vi "SystemeinstellungenV2_Screenshots.vi"(8 "error in":errorcluster, 11 "Screenshots Pfad":path) -> (0 "error out 2":errorcluster caption="error out", 3 "Screenshots Pfad  2":path caption="Screenshots Pfad")   [LabVIEW 2020, in "Backup.lvlib"]
uses:
  Backup.lvlib
  Seiten/System Einstellungen V2/System und Gaseinstellung V2.vi
  Seiten/System Einstellungen V2/System Einstellungen V2.lvlib
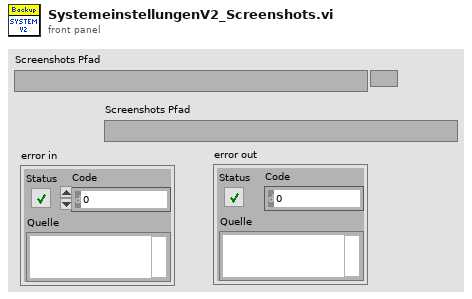
[diagram p1: front panel]
types:
  T1 = enum32{"Bad", "Idle", "Run top level", "Running"}
  T2 = typedef "imagedata.ctl" = cluster{"image type":i32, "image depth":i32, "image":u8[], "mask":u8[], "colors":u32[], "Rectangle":cluster{"left":i16, "top":i16, "right":i16, "bottom":i16}}
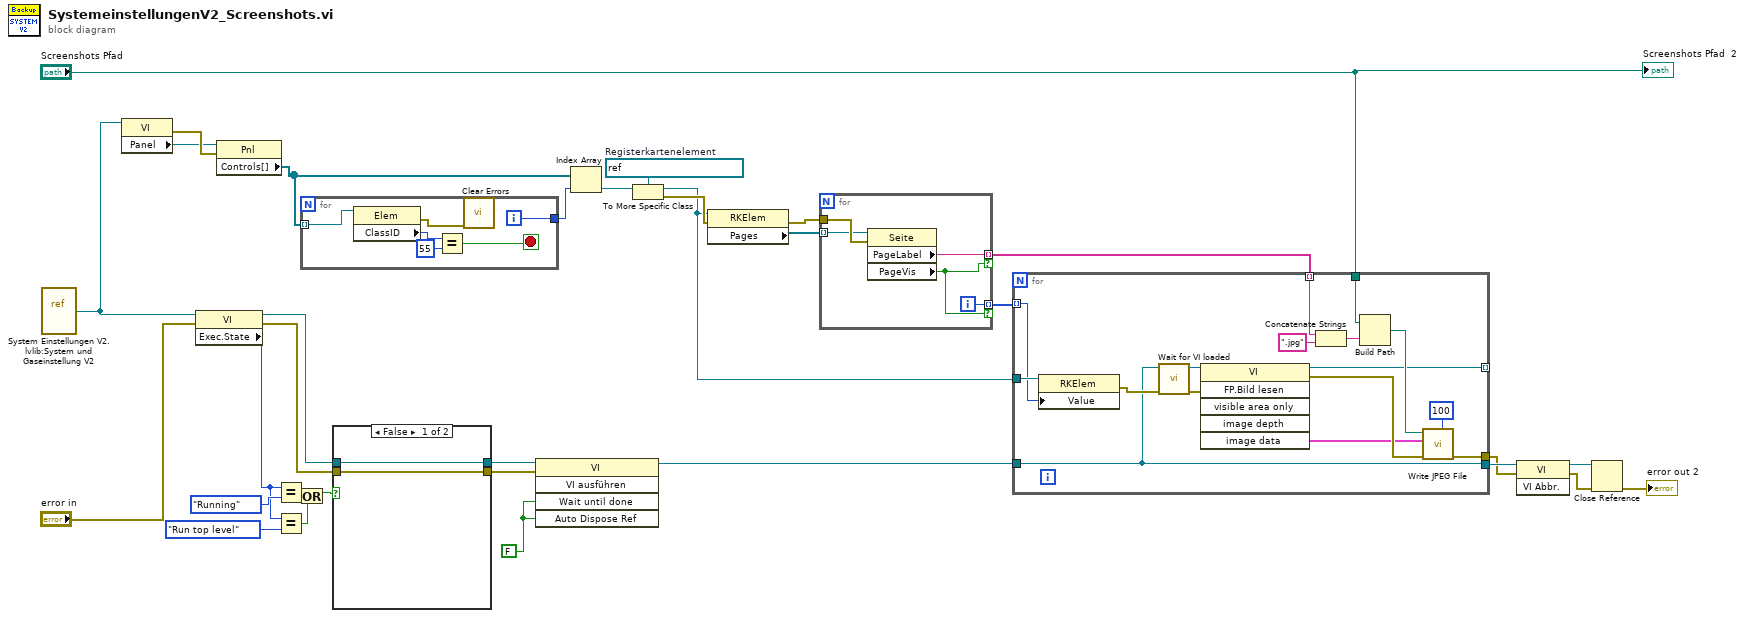
[diagram p0: block diagram]
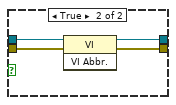
[diagram p2: hidden frame]
diagram:
  w18 = refnum<vi> refnum  # Registerkartenelement
  w30 = FALSE
  n1 = vi-ref "System Einstellungen V2.lvlib:System und Gaseinstellung V2.vi"() -> (w7:refnum<vi>)
  n2 = property class="VI"(reference=w7) -> (error out=w20:errorcluster, "Panel"=w19:refnum<vi>)  [unwired: 1 in, 1 out]
  n3 = property class="VI"(reference=w7, error in="error in") -> (reference out=w29:refnum<vi>, error out=w26:errorcluster, "Exec.State"=w23:T1)
  n4 = property class="Pnl"(reference=w19, error in=w20) -> ("Controls[]"=w3:refnum<vi>[])  [unwired: 2 out]
  n5 = Equal?(x=w23, y=T1."Running" ("Ausführung:Status")) -> (x = y?=w27:bool)
  n6 = Equal?(x=w23, y=T1."Run top level" ("Ausführung:Status")) -> (x = y?=w21:bool)
  n7 = Or(x=w27, y=w21) -> (x .or. y?=w22:bool)
  n8 = for {
    tunnel: w3 -> [w38] mode=indexing
    tunnel: [w34] -> w1
    i -> [w34]
    stop <- w35 stop-if-true
    n9 = property class="Elem"(reference=w38) -> (error out=w33:errorcluster, "ClassID"=w37:u32)  [unwired: 1 in, 1 out]
    n10 = Equal?(x=w37, y=u32 55) -> (x = y?=w35:bool)
    n11 = call <vilib>:"Clear Errors.vi"("error in (no error)"=w33) -> ()  [unwired: 5 in, 2 out]
  }
  n12 = case shown="False" w22 {
    tunnel: w29 -> [w40 w44]
    tunnel: [w40 w43] -> w28
    tunnel: w26 -> [w39 w42]
    tunnel: [w39 w41] -> w25
    frame False {
    }
    frame True {
      n13 = invoke class="VI" method="VI Abbr."(reference=w44, error in=w42) -> (reference out=w43:refnum<vi>, error out=w41:errorcluster)  [unwired: 1 in, 1 out]
    }
  }
  n14 = invoke class="VI" method="VI ausführen"(reference=w28, error in=w25, "Wait until done"=w30, "Auto Dispose Ref"=w30) -> (reference out=w6:refnum<vi>)  [unwired: 1 in, 4 out]
  n15 = Index Array(array=w3, index=w1) -> (element=w2:refnum<vi>)
  n16 = To More Specific Class(target class=w18, reference=w2) -> (specific class reference=w13:refnum<vi>, error out=w17:errorcluster)  [unwired: 1 in]
  n17 = property class="RKElem"(reference=w13, error in=w17) -> (error out=w16:errorcluster, "Pages"=w15:refnum<vi>[])  [unwired: 1 out]
  n18 = for {
    tunnel: w16 -> [w49]
    tunnel: w15 -> [w48] mode=indexing
    tunnel: [w47] -> w14 mode=indexing if=w45
    tunnel: [w46] -> w8 mode=indexing if=w45
    i -> [w46]
    n19 = property class="Seite"(reference=w48, error in=w49) -> ("PageLabel"=w47:string, "PageVis"=w45:bool)  [unwired: 2 out]
  }
  n20 = for {
    tunnel: [w57] -> _ mode=indexing
    tunnel: w14 -> [w56] mode=indexing
    tunnel: [w55] -> w10
    tunnel: w13 -> [w54]
    tunnel: w6 -> [w52]
    tunnel: [w52] -> w11
    tunnel: "Screenshots Pfad" -> [w51]
    tunnel: w8 -> [w50] mode=indexing
    n21 = property class="RKElem"(reference=w54, "Value"=w50) -> (error out=w53:errorcluster)  [unwired: 1 in, 1 out]
    n22 = call "Wait for VI loaded.vi"("error in"=w53, "VI Referenz"=w52) -> ("error out"=w65:errorcluster, "VI Referenz out"=w64:refnum<vi>)  [unwired: 7 in, 1 out]
    n23 = invoke class="VI" method="FP.Bild lesen"(reference=w64, error in=w65) -> (reference out=w57:refnum<vi>, error out=w59:errorcluster, "image data"=w58:T2)  [unwired: 4 in, 3 out]
    n24 = Concatenate Strings(w56, ".jpg" ("String")) -> (w62:string)
    n25 = Build Path(base path=w51, name or relative path=w62) -> (appended path=w61:path)
    n26 = call <vilib>:"Write JPEG File.vi"("quality (80)"=100, "error in (no error)"=w59, "image data"=w58, "path to JPEG file"=w61) -> ("error out"=w55:errorcluster)  [unwired: 6 in, 1 out]
  }
  n27 = invoke class="VI" method="VI Abbr."(reference=w11, error in=w10) -> (reference out=w12:refnum<vi>, error out=w5:errorcluster)  [unwired: 1 in, 1 out]
  n28 = Close Reference(reference=w12, error in (no error)=w5) -> (error out=→"error out 2":errorcluster)
  "Screenshots Pfad  2" <- "Screenshots Pfad"
